vi "PSHet_DAQ_SPhi_realtime.vi"() -> ()   [LabVIEW 2021]
uses:
  <vilib>/Analysis/1siggen.llb/Ramp Pattern by Samples.vi
  <vilib>/Analysis/NI_AALBase.lvlib
panel:
  in  "1st sideband offset":dbl
  in  "Phase offset":dbl
  out "PSHet phase v. time":cluster{dbl[], dbl[]}(graph)
  in  "Record Length":dbl=20.0
  in  "Sideband factor":dbl=1.0 format="%_3f"
  in  "N Samples":dbl=100.0
  in  "Sampling Rate":dbl=1000.0
  out "PSHet amplitude v. time":cluster{dbl[], dbl[]}[](graph)
  in  "Stop":bool
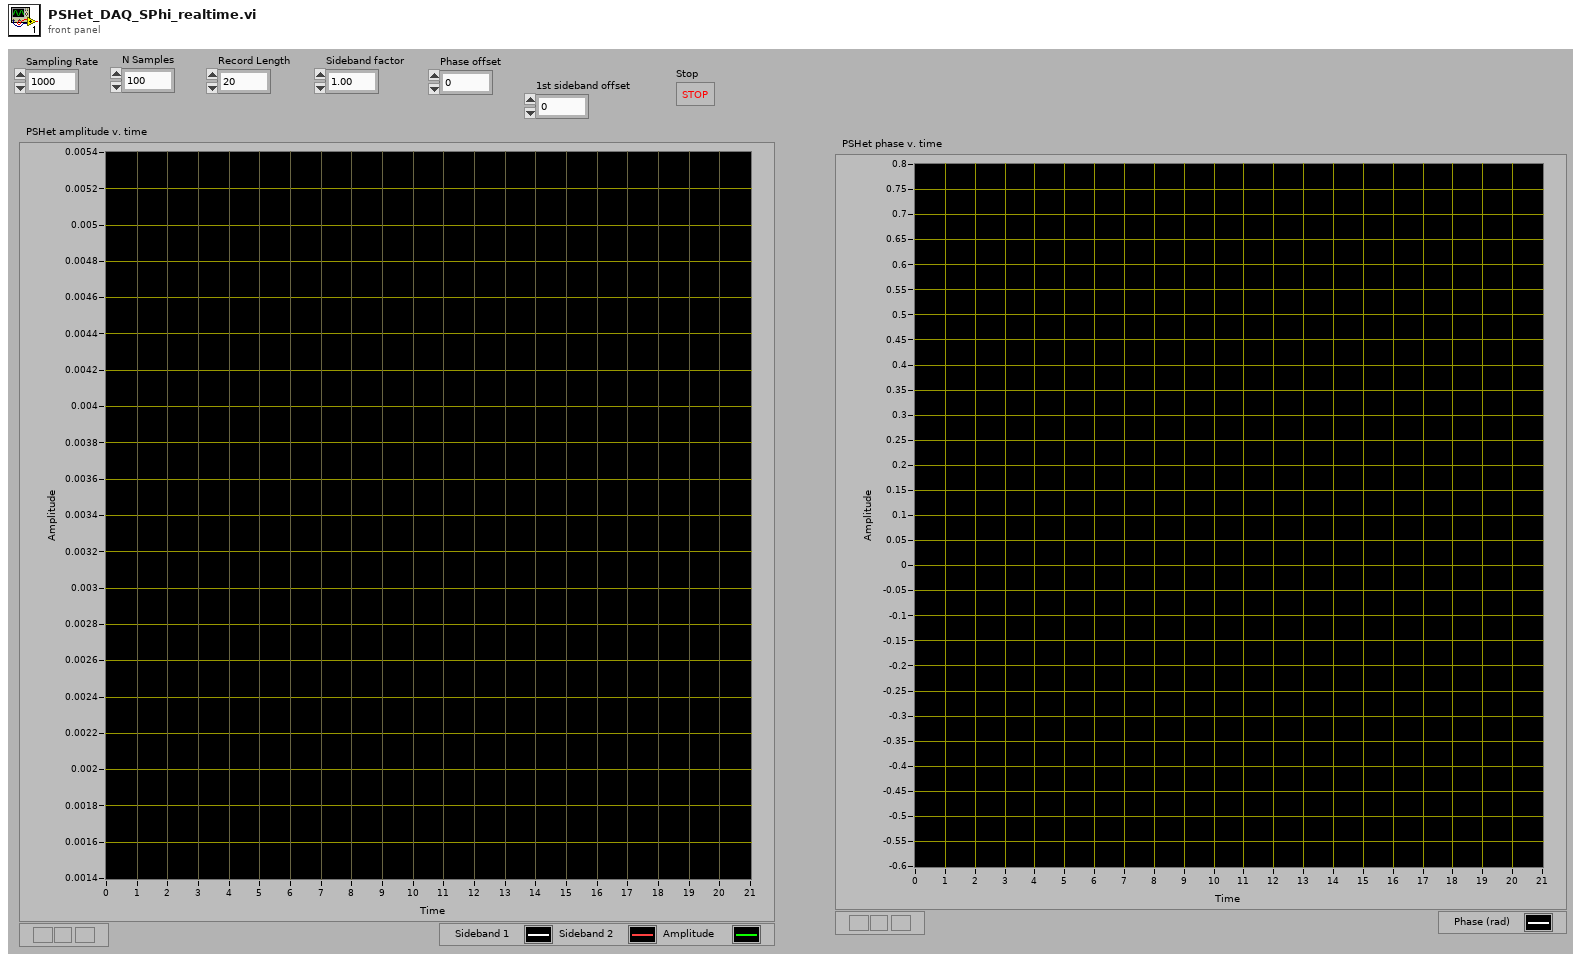
[diagram p1: front panel]
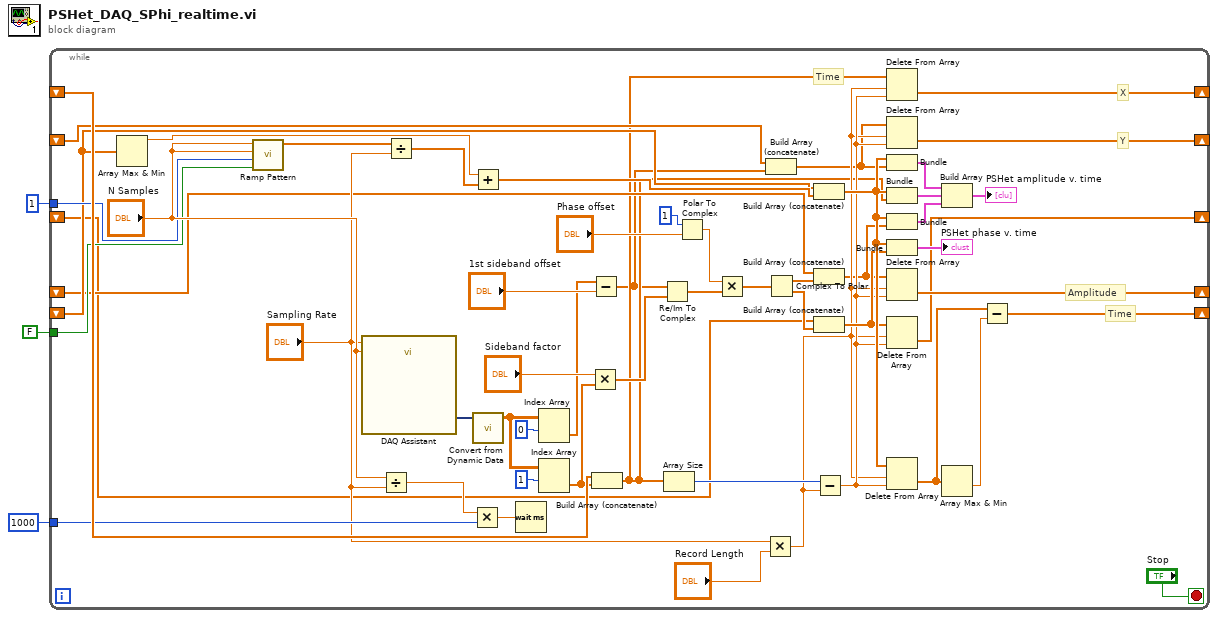
[diagram p0: block diagram]
diagram:
  n1 = while {
    shift-right: [w38] -> _
    shift-left: _ -> [w57]
    shift-right: [w37] -> _
    shift-left: _ -> [w56]
    tunnel: 1000 -> [w50]
    shift-right: [w36] -> _
    shift-left: _ -> [w14]
    tunnel: 1 -> [w45]
    tunnel: FALSE -> [w44]
    shift-right: [w12] -> _
    shift-left: _ -> [w32]
    shift-right: [w27] -> _
    shift-left: _ -> [w13]
    stop <- "Stop" stop-if-true
    # "Amplitude"
    # "Time"
    # "Y"
    # "X"
    # "Time"
    n2 = Array Max & Min(array=w32) -> (max value=w41:dbl)  [unwired: 3 out]
    n3 = call-poly <vilib>:"Ramp Pattern.vi"("exclude end?"=w44, "start"=w45, "end"="N Samples", "samples"="N Samples") -> ("Ramp Pattern"=w35:dbl[])  [unwired: 6 in, 1 out]
    n4 = call "DAQ Assistant"("rate"="Sampling Rate", "number of samples"="N Samples") -> ("data"=w52:dynamicdata)  [unwired: 15 in, 2 out]
    n5 = Divide(x="N Samples", y="Sampling Rate") -> (x/y=w43:dbl)
    n6 = Divide(x=w35, y="Sampling Rate") -> (x/y=w34:dbl[])
    n7 = Multiply(x=w43, y=w50) -> (x*y=w49:dbl)
    n8 = Add(x=w41, y=w34) -> (x+y=w42:dbl[])
    n9 = call "Convert from Dynamic Data"("Dynamic Data Type"=w52) -> ("Array"=w47:dbl[][])  [unwired: 3 in]
    n10 = Wait (ms)(milliseconds to wait=w49) -> ()  [unwired: 1 out]
    n11 = Index Array(array=w47, index (row)=0) -> (element=w5:dbl[])  [unwired: 1 in]
    n12 = Index Array(array=w47, index (row)=1) -> (element=w29:dbl[])  [unwired: 1 in]
    n13 = Multiply(x="Sideband factor", y=w29) -> (x*y=w23:dbl[])
    n14 = Subtract(x=w5, y="1st sideband offset") -> (x-y=w4:dbl[])
    n15 = Build Array (concatenate)(w57, w29) -> (w9:dbl[])
    n16 = Re/Im To Complex(1:w23, 2:w4) -> (0:w16:cdb[])
    n17 = Array Size(array=w9) -> (size(s)=w39:i32)
    n18 = Polar To Complex(1:"Phase offset", 2:1) -> (0:w17:cdb)
    n19 = Multiply(x=w17, y=w16) -> (x*y=w18:cdb[])
    n20 = Multiply(x="Sampling Rate", y="Record Length") -> (x*y=w24:dbl)
    n21 = Build Array (concatenate)(w56, w4) -> (w6:dbl[])
    n22 = Complex To Polar(r * e^(i*theta)=w18) -> (r=w19:dbl[], theta=w21:dbl[])
    n23 = Build Array (concatenate)(w32, w42) -> (w30:dbl[])
    n24 = Build Array (concatenate)(w14, w19) -> (w8:dbl[])
    n25 = Build Array (concatenate)(w13, w21) -> (w26:dbl[])
    n26 = Subtract(x=w39, y=w24) -> (x-y=w25:dbl)
    n27 = Delete From Array(array=w9, length=w24, index=w25) -> (deleted portion=w38:dbl[])  [unwired: 1 out]
    n28 = Delete From Array(array=w6, length=w24, index=w25) -> (deleted portion=w37:dbl[])  [unwired: 1 out]
    n29 = Bundle(w30, w6) -> (w55:cluster{dbl[], dbl[]})  [unwired: 1 in]
    n30 = Bundle(w30, w9) -> (w54:cluster{dbl[], dbl[]})  [unwired: 1 in]
    n31 = Bundle(w30, w8) -> (w15:cluster{dbl[], dbl[]})  [unwired: 1 in]
    n32 = Bundle(w30, w26) -> (→"PSHet phase v. time":cluster{dbl[], dbl[]})  [unwired: 1 in]
    n33 = Delete From Array(array=w8, length=w24, index=w25) -> (deleted portion=w36:dbl[])  [unwired: 1 out]
    n34 = Delete From Array(array=w26, length=w24, index=w25) -> (deleted portion=w27:dbl[])  [unwired: 1 out]
    n35 = Delete From Array(array=w30, length=w24, index=w25) -> (deleted portion=w10:dbl[])  [unwired: 1 out]
    n36 = Build Array(w55, w54, w15) -> (→"PSHet amplitude v. time":cluster{dbl[], dbl[]}[])
    n37 = Array Max & Min(array=w10) -> (min value=w11:dbl)  [unwired: 3 out]
    n38 = Subtract(x=w10, y=w11) -> (x-y=w12:dbl[])
  }
